vi "SendMessageToClient.vi"(8 "error in (no error)":errorcluster, 10 "Message":string, 11 "TCP_Client_Window in":refnum<class "TCP_Client_Window.lvclass">) -> (0 "error out":errorcluster, 3 "TCP_Client_Window out":refnum<class "TCP_Client_Window.lvclass">)   [LabVIEW 2023, in "TCP_Client_Window.lvlib" / "TCP_Client_Window.lvclass"]
uses:
  TCP_Client_Window.lvclass
  <vilib>/ActorFramework/Actor/Actor.lvclass/Actor.ctl
  TCP_Client_Window.lvclass/TCP_Client_Window.ctl
  TCP_ClientWindow_Controller Messages/NewMessageToSend Msg/NewMessageToSend Msg.lvclass/NewMessageToSend Msg.ctl
  <vilib>/ActorFramework/Message Enqueuer/Message Enqueuer.lvclass/Message Enqueuer.ctl
  <vilib>/ActorFramework/Message Enqueuer/Enqueue.vi
  TCP_ClientWindow_Controller Messages/NewMessageToSend Msg/NewMessageToSend Msg.lvclass
  <vilib>/ActorFramework/Message Priority Queue/Priority Enqueue.vi
  <vilib>/ActorFramework/Actor/Actor.lvclass
  TCP_Server_Connection_Handler/TypeDefinitions/messageType.ctl
  TCP_Server_Connection_Handler/TCP_Server_Connection_Handler.lvlib
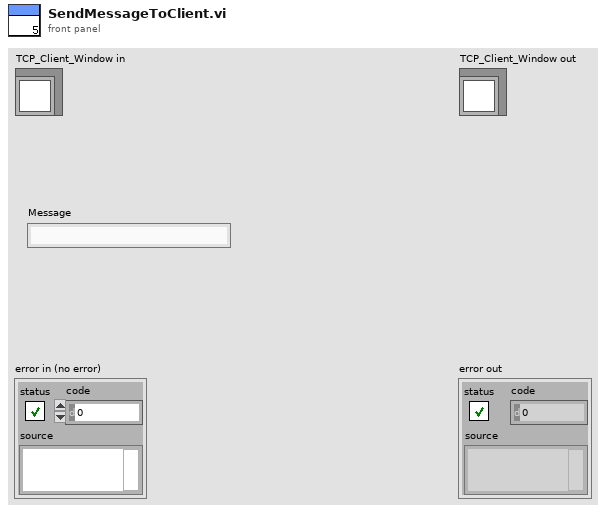
[diagram p1: front panel]
types:
  T1 = typedef "TCP_Server_Connection_Handler.lvlib/messageType.ctl" = enum16{"message", "file", "get", "ShutDown"}
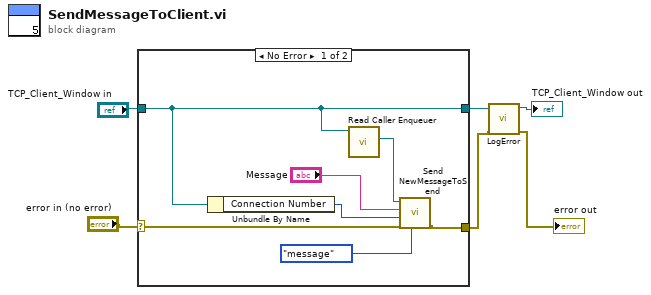
[diagram p0: block diagram]
diagram:
  n1 = case shown="No Error" "error in (no error)" {
    selector: "error in (no error)" -> [w9 w15]
    tunnel: [w8 w15] -> w2
    tunnel: [w11 w14] -> w4
    tunnel: "TCP_Client_Window in" -> [w11 w14]
    frame No Error {
      n2 = Unbundle By Name(w11) -> ("Connection Number"=w13:i32)
      n3 = call <vilib>:"Read Caller Enqueuer.vi"("Actor"=w11) -> ("Caller Enqueuer"=w10:refnum<class "Message Enqueuer.lvclass">)  [unwired: 10 in]
      n4 = call "Send NewMessageToSend.vi"("MessageType"=messageType."message", "error in (no error)"=w9, "Connection Number"=w13, "Message"="Message", "Message Enqueuer"=w10) -> ("error out"=w8:errorcluster)  [unwired: 5 in, 1 out]
    }
    frame Error {
    }
  }
  n5 = call "LogError.vi"("error in (no error)"=w2, "TCP_Client_Window in"=w4) -> ("error out"=→"error out":errorcluster, "TCP_Client_Window out"=→"TCP_Client_Window out":refnum<class "TCP_Client_Window.lvclass">)  [unwired: 8 in]
